vi "add tag select.vi"(8 "error in":errorcluster, 9 "data type":T1=enum."Boolean", 10 "tag select name":string, 11 "tag select module configuration in":refnum<class "tag select module configuration.lvclass">) -> (0 "error out":errorcluster, 2 "created channels":refnum<class "TBM channel.lvclass">[](array[class]), 3 "tag select module configuration out":refnum<class "tag select module configuration.lvclass">)   [LabVIEW 2013, in "tag select module configuration.lvclass"]
uses:
  tag select module configuration.lvclass
  <vilib>/NI/Tag Bus Module Framework/channel/TBM channel.lvclass
  <vilib>/NI/Tag Bus/tag/Data Type.ctl
  tag select module configuration.lvclass/tag select module configuration.ctl
  tag select configuration.ctl
  <vilib>/NI/Tag Bus/tag/tag descriptor.lvclass
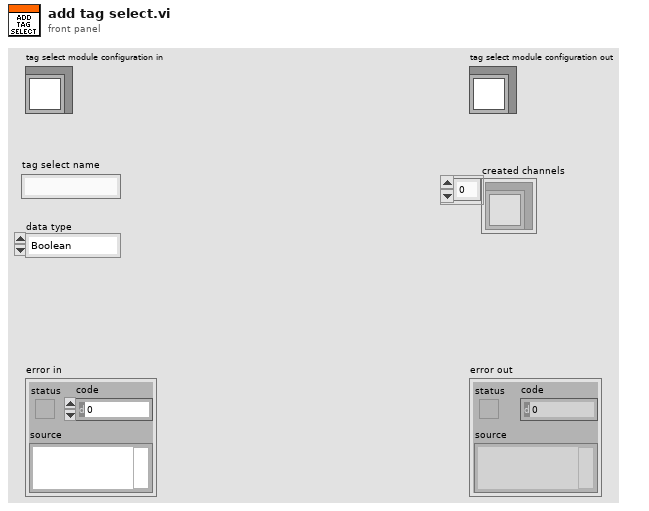
[diagram p1: front panel]
types:
  T1 = typedef "tag bus.lvlib/tag descriptor.lvclass/Data Type.ctl" = enum16{"Double", "Single", "I64", "I32", "I16", "I8", "U64", "U32", "U16", "U8", "Boolean", "String", "Array of Double", "Array of Single", "Array of I64", "Array of I32", "Array of I16", "Array of I8", "Array of U64", "Array of U32", "Array of U16", "Array of U8", "Array of Boolean", "Array of String"}
  T2 = typedef "tag select module configuration.lvclass/tag select configuration.ctl" = cluster{"tag select name":string, "data type":T1, "output":refnum<class "TBM channel.lvclass">, "select":refnum<class "TBM channel.lvclass">, "input channels":refnum<class "TBM channel.lvclass">[]}
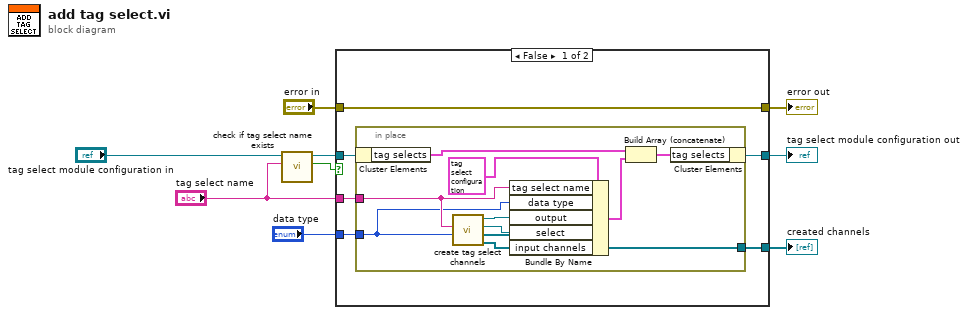
[diagram p0: block diagram]
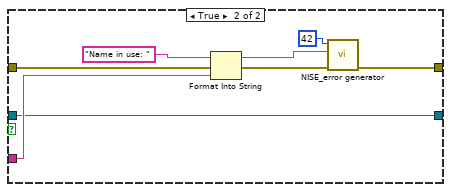
[diagram p2: hidden frame]
diagram:
  n1 = call "check if tag select name exists.vi"("name to locate"="tag select name", "tag select module configuration in"="tag select module configuration in") -> ("found?"=w6:bool, "tag select module configuration out"=w4:refnum<class "tag select module configuration.lvclass">)  [unwired: 6 in, 2 out]
  n2 = case shown="False" w6 {
    tunnel: [w13 w32] -> w8
    tunnel: "error in" -> [w13 w33]
    tunnel: "tag select name" -> [w12 w28]
    tunnel: [w14 w26] -> w5
    tunnel: w4 -> [w15 w26]
    tunnel: [w11 _] -> w3
    tunnel: "data type" -> [w10 _]
    frame False {
      n3 = in-place {
        in-place-border: w12 -> [w19]
        in-place-border: [w17] -> w11
        in-place-border: w10 -> [w16]
        n4 = in-place-cluster #1(w15) -> ("tag selects"=w25:T2[])
        n5 = call "create tag select channels.vi"("data type"=w16, "tag select name"=w19) -> ("created channels"=w17:refnum<class "TBM channel.lvclass">[], "inputs"=w18:refnum<class "TBM channel.lvclass">[], "select"=w20:refnum<class "TBM channel.lvclass">, "output"=w21:refnum<class "TBM channel.lvclass">)  [unwired: 6 in]
        n6 = Bundle By Name(cluster=T2 {"tag select name"="", "data type"=enum."Double", "output"=refnum, "select"=refnum, "input channels"=[]} ("alarm config"), "tag select name"=w19, "data type"=w16, "output"=w21, "select"=w20, "input channels"=w18) -> (w22:T2)
        n7 = Build Array (concatenate)(w25, w22) -> (w24:T2[])
        n8 = in-place-cluster #1("tag selects"=w24) -> (w14:refnum<class "tag select module configuration.lvclass">)
      }
    }
    frame True {
      n9 = Format Into String(initial string="Name in use: " ("append error message"), error in=w33, w28) -> (resulting string=w27:string, error out=w30:errorcluster)  [unwired: 1 in]
      n10 = call <vilib>:"NISE_error generator.vi"("error in"=w30, "append error message"=w27, "error code (0)"=42) -> ("error out"=w32:errorcluster)  [unwired: 6 in]
    }
  }
  "error out" <- w8
  "tag select module configuration out" <- w5
  "created channels" <- w3
